vi "stopAllMotion.vi"(8 "error in (no error)":errorcluster, 11 "SpectrographClientCommunicator in":refnum<class "SpectrographClientCommunicator.lvclass">) -> (0 "error out":errorcluster, 3 "SpectrographClientCommunicator out":refnum<class "SpectrographClientCommunicator.lvclass">)   [LabVIEW 2016, in "SpectrographClientCommunicator.lvclass"]
uses:
  SpectrographClientCommunicator.lvclass
  SpectrographTypeDef/SpectrographCMDs.ctl
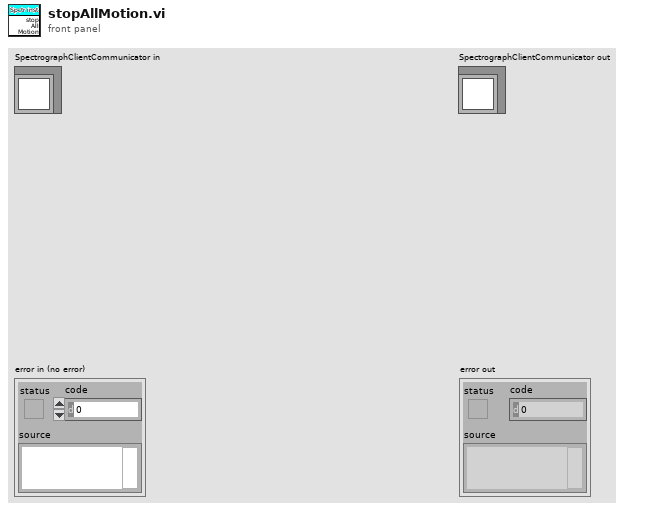
[diagram p1: front panel]
types:
  T1 = typedef "SpectrographCMDs.ctl" = enum16{"getFilterWheelPosition", "getGratingWheelPosition", "moveLinearStage", "moveGratingWheel", "moveFilterWheel", "homeLinearStage", "getLinearStageStatus", "getGratingWheelStatus", "getFilterWheelStatus", "stopAllMotion"}
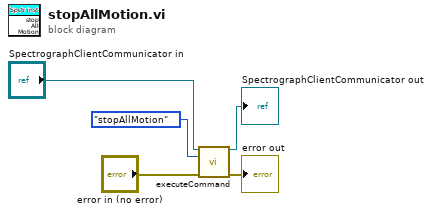
[diagram p0: block diagram]
diagram:
  n1 = call "executeCommand.vi"("SpectrographClientCommunicator in"="SpectrographClientCommunicator in", "Command"=SpectrographCMDs."stopAllMotion", "error in (no error)"="error in (no error)") -> ("SpectrographClientCommunicator out"=→"SpectrographClientCommunicator out":refnum<class "SpectrographClientCommunicator.lvclass">, "error out"=→"error out":errorcluster)  [unwired: 8 in, 3 out]
